vi "Alle_Sensoren.vi"() -> (1 "Array":dbl[](array[numeric]))   [LabVIEW 2016]
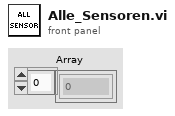
[diagram p1: front panel]
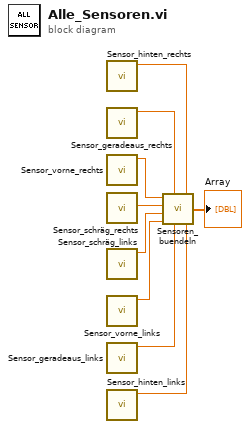
[diagram p0: block diagram]
diagram:
  n1 = call "Sensor_hinten_rechts.vi"() -> ("hinten rechts"=w2:dbl)  [unwired: 11 in]
  n2 = call "Sensor_geradeaus_rechts.vi"() -> ("geradeaus rechts"=w3:dbl)  [unwired: 11 in]
  n3 = call "Sensor_vorne_rechts.vi"() -> ("vorne rechts"=w4:dbl)  [unwired: 11 in]
  n4 = call "Sensor_schräg_rechts.vi"() -> ("schräg rechts"=w1:dbl)  [unwired: 11 in]
  n5 = call "Sensor_schräg_links.vi"() -> ("schräg links"=w5:dbl)  [unwired: 11 in]
  n6 = call "Sensor_vorne_links.vi"() -> ("vorne links"=w6:dbl)  [unwired: 11 in]
  n7 = call "Sensor_geradeaus_links.vi"() -> ("geradeaus links"=w7:dbl)  [unwired: 11 in]
  n8 = call "Sensor_hinten_links.vi"() -> ("hinten links"=w8:dbl)  [unwired: 11 in]
  n9 = call "Sensoren_buendeln.vi"("rechts seite"=w4, "rechts geradeaus"=w3, "rechts Schräg"=w1, "Links schräg"=w5, "Links Geradeaus"=w7, "Links seite"=w6, "rechts hinten"=w2, "links hinten"=w8) -> ("SensorArray"=→"Array":dbl[])
